vi "CLD 1 Elapsed Time Express Front Panel.vi"() -> ()   [LabVIEW 2019]
doc: "LabVIEW CLD 1 Exercise"
panel:
  out "error out":errorcluster
  in  "error in":errorcluster
  out "Elapsed Time":string
  out "Time has Elapsed":bool
  in  "Auto Reset":bool=TRUE
  in  "Reset Button":bool
  in  "Stop VI":bool
  in  "Time Target (s)":dbl
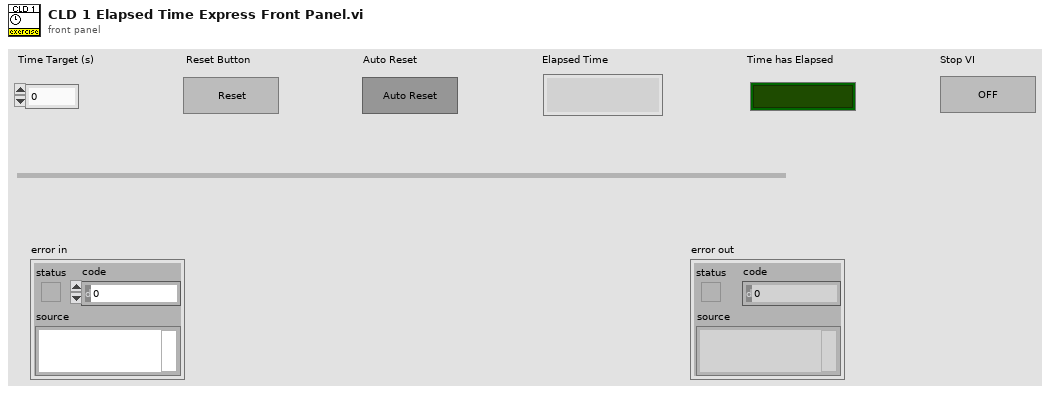
[diagram p1: front panel]
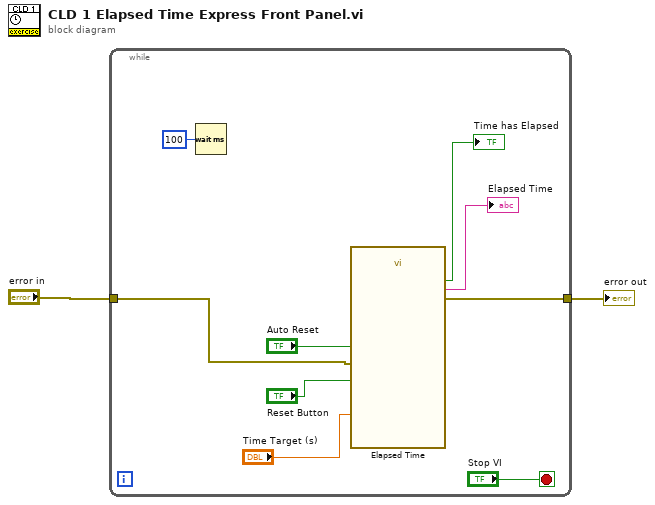
[diagram p0: block diagram]
diagram:
  n1 = while {
    tunnel: "error in" -> [w6]
    tunnel: [w5] -> w1
    stop <- "Stop VI" stop-if-true
    n2 = Wait (ms)(milliseconds to wait=u32 100) -> ()  [unwired: 1 out]
    n3 = call "Elapsed Time"("Time Target (s)"="Time Target (s)", "Reset"="Reset Button", "Auto Reset"="Auto Reset", "error in (no error)"=w6) -> ("Time has Elapsed"=→"Time has Elapsed":bool, "Elapsed Time Text"=→"Elapsed Time":string, "error out"=w5:errorcluster)  [unwired: 8 in, 5 out]
  }
  "error out" <- w1
